vi "Snap to bottom (centered).vi"(1 "Large Rect":T1, 2 "Small Rect":T1) -> (0 "Snapped to bottom center":T1)   [LabVIEW 2012]
doc: "This VI calculates the position of a snapped-to-bottom rectangle from the positions of a large rectangle and a smaller one that will be positioned inside."
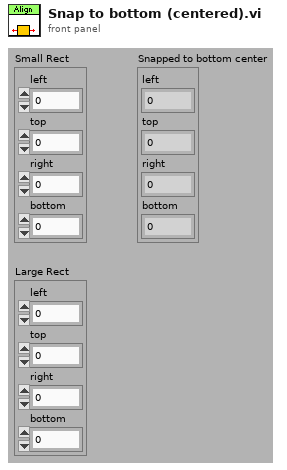
[diagram p1: front panel]
types:
  T1 = cluster{"left":i16, "top":i16, "right":i16, "bottom":i16}
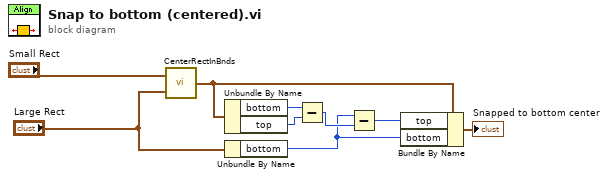
[diagram p0: block diagram]
diagram:
  n1 = call <vilib>:"CenterRectInBnds.vi"("bounds"="Large Rect", "rect"="Small Rect") -> ("centered rect"=w1:T1)
  n2 = Unbundle By Name(w1) -> ("bottom"=w4:i16, "top"=w5:i16)
  n3 = Unbundle By Name("Large Rect") -> ("bottom"=w3:i16)
  n4 = Subtract(x=w4, y=w5) -> (x-y=w6:i16)
  n5 = Subtract(x=w3, y=w6) -> (x-y=w2:i16)
  n6 = Bundle By Name(cluster=w1, "top"=w2, "bottom"=w3) -> (→"Snapped to bottom center":T1)
